vi "GPIB with VISA functions.vi"() -> ()   [LabVIEW 2023]
doc: "This example requires NI-488.2 and NI-VISA to be installed on the system. The example shows how to communicate with a GPIB instrument using VISA reads, writes, and formatting functions on the returned data. This example will work using an NI Instrument Simulator or other instrument that has similar behavior."
panel:
  in  "Waveform":enum16{"SIN", "SQU", "RAND"}(ring)
  out "Waveform Graph":dbl[](graph)
  out "Raw Data":string
  in  "VISA GPIB Resource":refnum<visa-resource-name>="GPIB0::2::INSTR"
  # "Overview: Demonstrates the use of the VISA functions to communicate to a GPIB instrument.\nRequirements: NI-488.2 and NI-VISA Drivers\nInstructions:\n1. Ensure the resource specified in the VISA GPIB Resource control is properly configured in Measurement & Automation Explorer.\n2. Run the VI.\n3. If your instrument recognizes the \"SOUR:FUNC\" and \"SENS:DATA?\" commands, it should return the specified Waveform data."
  # "On Windows/Linux, consider using the Instrument Driver Finder (Help > Find Instrument Drivers) to search for an instrument driver for your instrument."
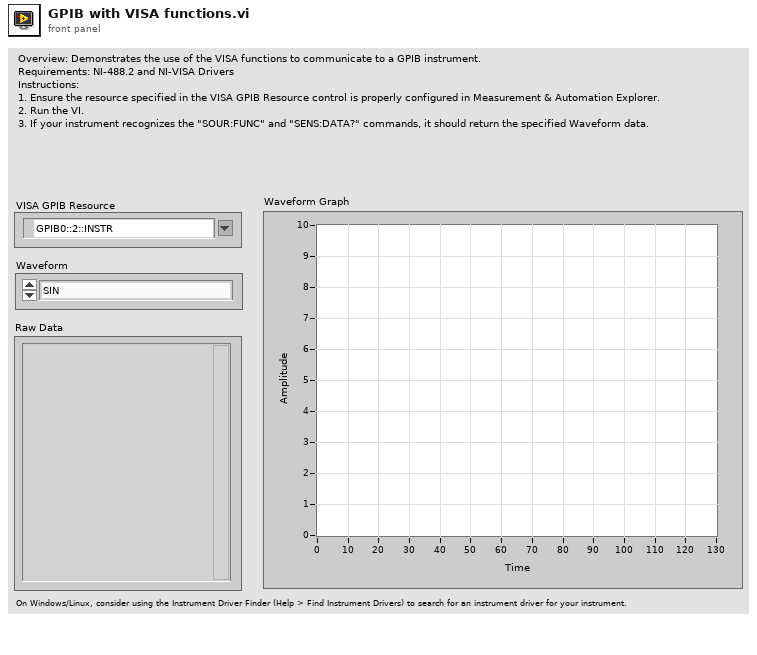
[diagram p1: front panel]
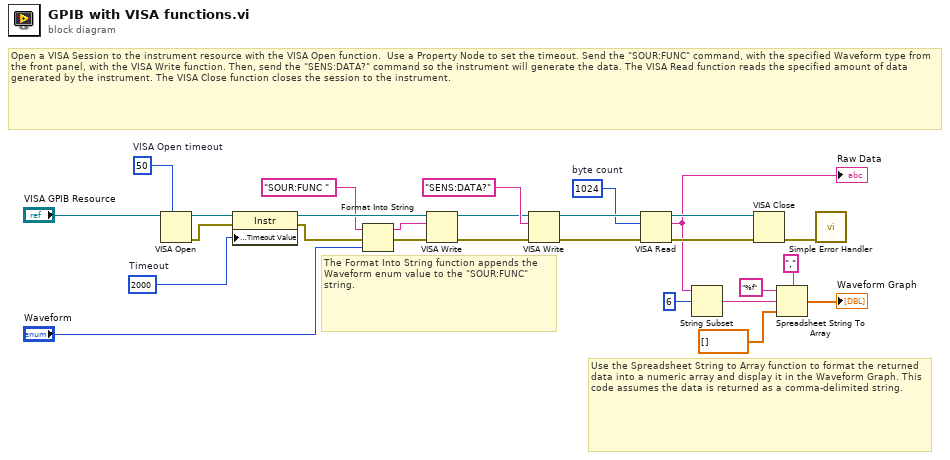
[diagram p0: block diagram]
diagram:
  w17 = u32 1024  # byte count
  w22 = u32 2000  # Timeout
  w23 = u32 50  # VISA Open timeout
  # "Use the Spreadsheet String to Array function to format the returned data into a numeric array and display it in the Waveform Graph. This code assumes the data is returned as a comma-delimited string."
  # "The Format Into String function appends the Waveform enum value to the \"SOUR:FUNC\" string."
  # "Open a VISA Session to the instrument resource with the VISA Open function.  Use a Property Node to set the timeout. Send the \"SOUR:FUNC\" command, with the specified Waveform type from the front panel, with the VISA Write function. Then, send the \"SENS:DATA?\" command so the instrument will generate the data. The VISA Read function reads the specified amount of data generated by the instrument. The VISA Close function closes the session to the instrument."
  n1 = VISA Open(timeout (0)=w23, VISA resource name="VISA GPIB Resource") -> (VISA resource name=w21:refnum<visa-resource-name>, error out=w20:errorcluster)  [unwired: 3 in]
  n2 = property class="Instr"(reference=w21, error in=w20, "General Settings:Timeout Value"=w22) -> (reference out=w8:refnum<visa-resource-name>, error out=w4:errorcluster)
  n3 = Format Into String(initial string="SOUR:FUNC " ("string"), error in=w4, "Waveform") -> (resulting string=w1:string, error out=w3:errorcluster)  [unwired: 1 in]
  n4 = VISA Write(VISA resource name=w8, write buffer=w1, error in (no error)=w3) -> (VISA resource name out=w7:refnum<visa-resource-name>, error out=w6:errorcluster)  [unwired: 1 out]
  n5 = VISA Write(VISA resource name=w7, write buffer="SENS:DATA?" ("Write Buffer"), error in (no error)=w6) -> (VISA resource name out=w27:refnum<visa-resource-name>, error out=w25:errorcluster)  [unwired: 1 out]
  n6 = VISA Read(VISA resource name=w27, byte count=w17, error in (no error)=w25) -> (VISA resource name out=w26:refnum<visa-resource-name>, read buffer=w15:string, error out=w24:errorcluster)  [unwired: 1 out]
  "Raw Data" <- w15
  n7 = String Subset(string=w15, offset (0)=6) -> (substring=w13:string)  [unwired: 1 in]
  n8 = VISA Close(VISA resource name=w26, error in (no error)=w24) -> (error out=w16:errorcluster)
  n9 = Spreadsheet String To Array(delimiter (Tab)=",", format string="%f", spreadsheet string=w13, array type (2D Dbl)=dbl[] []) -> (array=→"Waveform Graph":dbl[])
  n10 = call <vilib>:"Simple Error Handler.vi"("error in (no error)"=w16) -> ()  [unwired: 4 in, 5 out]
